vi "Create.vi"(6 "Labels":map{string, string}(c390), 7 "Registry Name":string="_default_registry", 8 "error in (no error)":errorcluster, 9 "Auto-Register? (T)":bool=TRUE, 11 "Volumes":path[](array[path])) -> (0 "error out":errorcluster, 3 "Disk Collector out":refnum<class "Disk Collector.lvclass">)   [LabVIEW 2020, in "Disk Collector.lvclass"]
uses:
  Disk Collector.lvclass
  C:/Program Files (x86)/National Instruments/LabVIEW 2020/vi.lib/TheLabVIEWLab/PromVIEW/collector/collectable/Collectable.lvclass
  Disk Collector.lvclass/Disk Collector.ctl
  <vilib>/TheLabVIEWLab/PromVIEW/metrics/gauge/Gauge.lvclass
  <vilib>/TheLabVIEWLab/PromVIEW/registry/session/Registry Session.lvclass
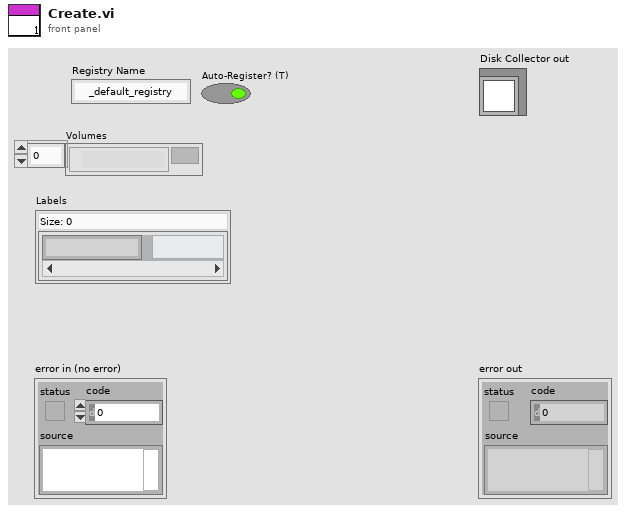
[diagram p1: front panel]
types:
  T1 = typedef "Registry.lvlib/Registry Session.lvclass/Session Handle.ctl" = refnum<data-value>
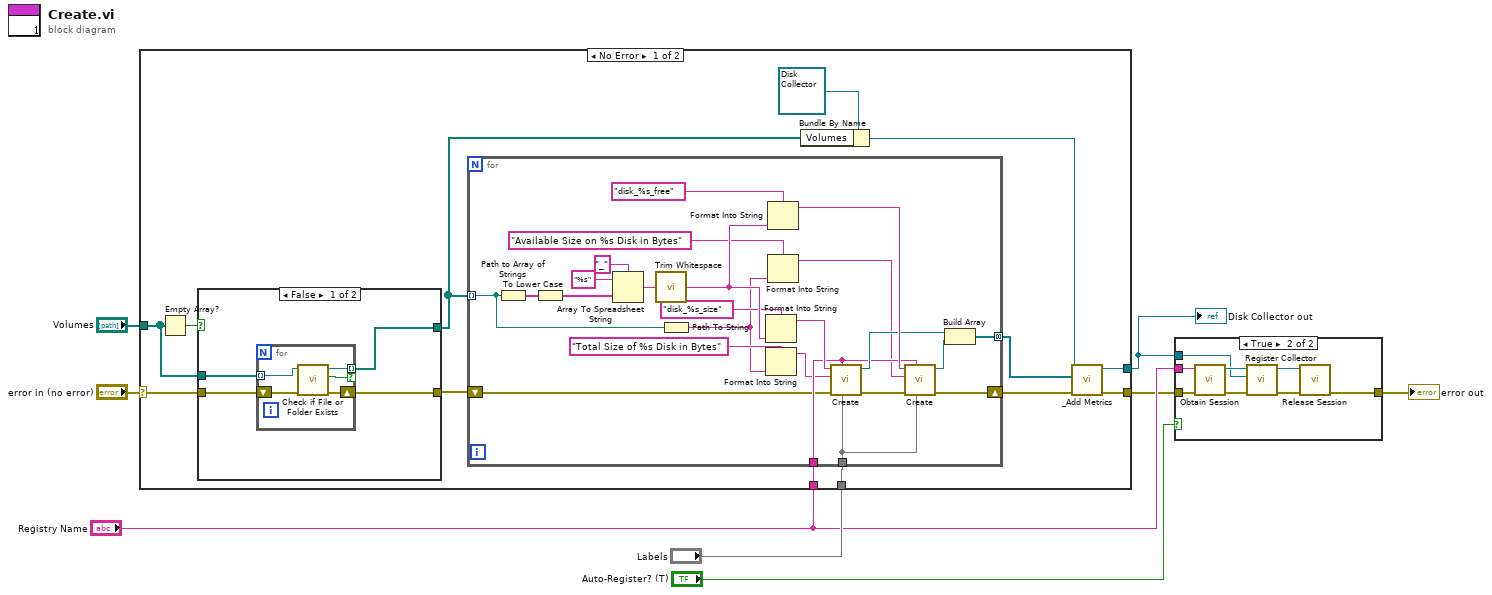
[diagram p0: block diagram]
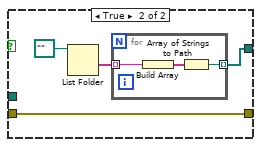
[diagram p3: hidden frame]
diagram:
  n1 = case shown="No Error" "error in (no error)" {
    selector: "error in (no error)" -> [w18 w62]
    tunnel: [w13 w62] -> w4
    tunnel: [w15 _] -> w3
    tunnel: "Volumes" -> [w19 _]
    tunnel: "Registry Name" -> [w12 _]
    tunnel: "Labels" -> [w11 _]
    frame No Error {
      n2 = Empty Array?(array=w19) -> (empty?=w20:bool)
      n3 = case shown="False" w20 {
        tunnel: w19 -> [w49 _]
        tunnel: [w48 w56] -> w16
        tunnel: w18 -> [w47 w55]
        tunnel: [w46 w55] -> w9
        frame False {
          n4 = for {
            tunnel: w49 -> [w54] mode=indexing
            tunnel: [w53] -> w48 mode=indexing if=w52
            shift-right: [w50] -> w46
            shift-left: w47 -> [w51]
            n5 = call <vilib>:"Check if File or Folder Exists.vi"("error in (no error)"=w51, "path"=w54) -> ("error out"=w50:errorcluster, "file or folder exists?"=w52:bool, "dup path"=w53:path)  [unwired: 7 in]
          }
        }
        frame True {
          n6 = List Folder(path=path "") -> (folder names=w57:string[])  [unwired: 3 in, 3 out]
          n7 = for {
            tunnel: w57 -> [w60] mode=indexing
            tunnel: [w61] -> w56 mode=indexing
            n8 = Build Array(w60) -> (w59:string[])
            n9 = Array of Strings to Path(0:w59) -> (2:w61:path)  [unwired: 1 in]
          }
        }
      }
      n10 = for {
        tunnel: w16 -> [w27] mode=indexing
        tunnel: [w34] -> w14 mode=concatenating
        tunnel: w12 -> [w33]
        tunnel: w11 -> [w32]
        shift-right: [w22] -> w10
        shift-left: w9 -> [w23]
        n11 = Path to Array of Strings(0:w27) -> (2:w29:string[])  [unwired: 1 out]
        n12 = To Lower Case(string=w29) -> (all lower case string=w28:string[])
        n13 = Array To Spreadsheet String(delimiter (Tab)="_", array=w28, 3:"%s" ("format string")) -> (spreadsheet string=w44:string)
        n14 = call <vilib>:"Trim Whitespace.vi"("string"=w44) -> ("trimmed string"=w45:string)  [unwired: 1 in]
        n15 = Path To String(path=w27) -> (string=w26:string)
        n16 = Format Into String(format string="disk_%s_size", w45) -> (resulting string=w39:string)  [unwired: 2 in, 1 out]
        n17 = Format Into String(format string="Total Size of %s Disk in Bytes", w26) -> (resulting string=w25:string)  [unwired: 2 in, 1 out]
        n18 = Format Into String(format string="disk_%s_free", w45) -> (resulting string=w38:string)  [unwired: 2 in, 1 out]
        n19 = Format Into String(format string="Available Size on %s Disk in Bytes", w26) -> (resulting string=w24:string)  [unwired: 2 in, 1 out]
        n20 = call <vilib>:"Create.vi"("Labels"=w32, "Registry Name"=w33, "error in (no error)"=w23, "Description"=w25, "Metric Name"=w39) -> ("error out"=w37:errorcluster, "Gauge Ref"=w35:refnum<data-value>)  [unwired: 5 in]
        n21 = call <vilib>:"Create.vi"("Labels"=w32, "Registry Name"=w33, "error in (no error)"=w37, "Description"=w24, "Metric Name"=w38) -> ("error out"=w22:errorcluster, "Gauge Ref"=w36:refnum<data-value>)  [unwired: 5 in]
        n22 = Build Array(w35, w36) -> (w34:refnum<data-value>[])
      }
      n23 = Bundle By Name(cluster=refnum<class "Disk Collector.lvclass"> refnum ("Disk Collector in"), "Volumes"=w16) -> (w21:refnum<class "Disk Collector.lvclass">)
      n24 = call-dynamic "_Add Metrics.vi"("error in (no error)"=w10, "Metrics"=w14, "Default Collector in"=w21) -> ("error out"=w13:errorcluster, "Default Collector out"=w15:refnum<class "Disk Collector.lvclass">)  [unwired: 7 in]
    }
    frame Error {
    }
  }
  "Disk Collector out" <- w3
  n25 = case shown="True" "Auto-Register? (T)" {
    tunnel: "Registry Name" -> [_ w71]
    tunnel: w4 -> [w63 w70]
    tunnel: w3 -> [_ w67]
    tunnel: [w63 w64] -> w1
    frame False {
    }
    frame True {
      n26 = call <vilib>:"Obtain Session.vi"("error in (no error)"=w70, "Session  Name ()"=w71) -> ("error out"=w69:errorcluster, "Session Handle"=w68:T1)  [unwired: 8 in]
      n27 = call <vilib>:"Register Collector.vi"("error in (no error)"=w69, "Collector"=w67, "Session Handle in"=w68) -> ("error out"=w66:errorcluster, "Session Handle out"=w65:T1)  [unwired: 7 in]
      n28 = call <vilib>:"Release Session.vi"("error in (no error)"=w66, "Session Handle"=w65) -> ("error out"=w64:errorcluster)  [unwired: 9 in]
    }
  }
  "error out" <- w1
